vi "Page_AddCalSet.vi"(8 "error in (no error)":errorcluster, 11 "Configuration Paths":T1) -> (0 "error out":errorcluster, 3 "Configuration Paths out":T1)   [LabVIEW 2010]
uses:
  Config cluster.ctl
panel:
  in  "Delete Stim Profile":bool
  in  "Delete":bool
  in  "Selected Calibration Files":i32(listbox)
  in  "Add Calib":bool
  out "System Configuration File":string
  in  "Cancel Button":bool
  in  "OK Button":bool
  in  "Calibration files":i32[](listbox)
  # "1) Select the \"Calibration\" files for this calibration set"
  # "Available Calibration Files"
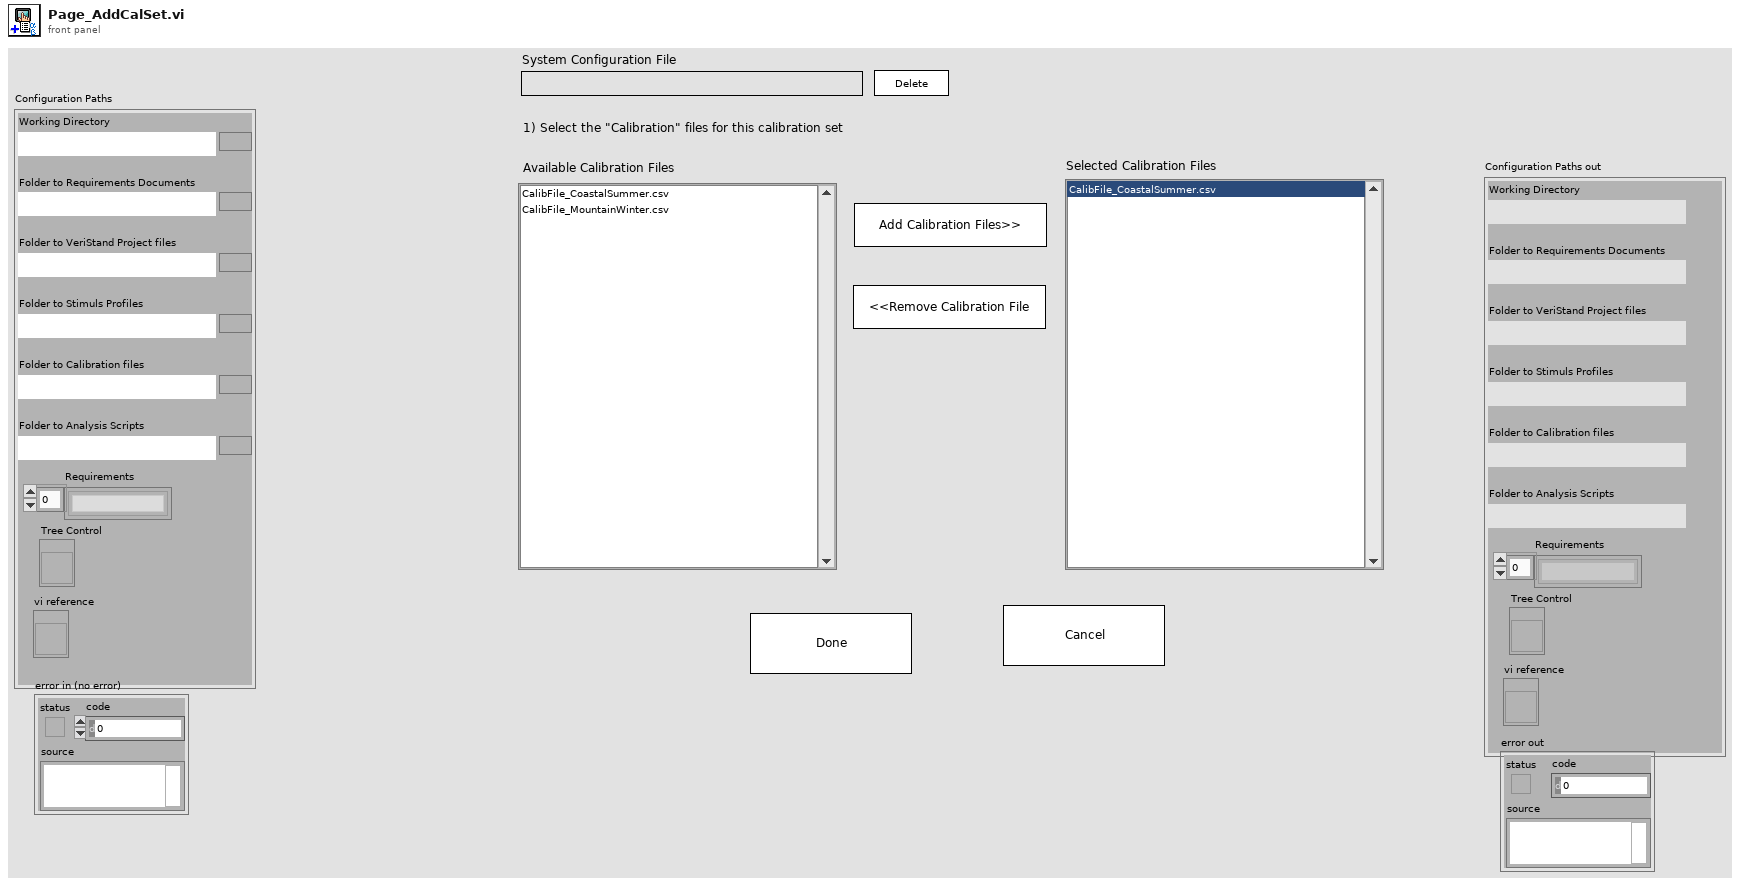
[diagram p1: front panel]
types:
  T1 = typedef "Config cluster.ctl" = cluster{"Working Directory":path, "Folder to Requirements Documents":path, "Folder to VeriStand Project files":path, "Folder to Stimuls Profiles":path, "Folder to Calibration files":path, "Folder to Analysis Scripts":path, "Requirements":string[], "Tree Control":refnum<vi>, "vi reference":refnum<vi>}
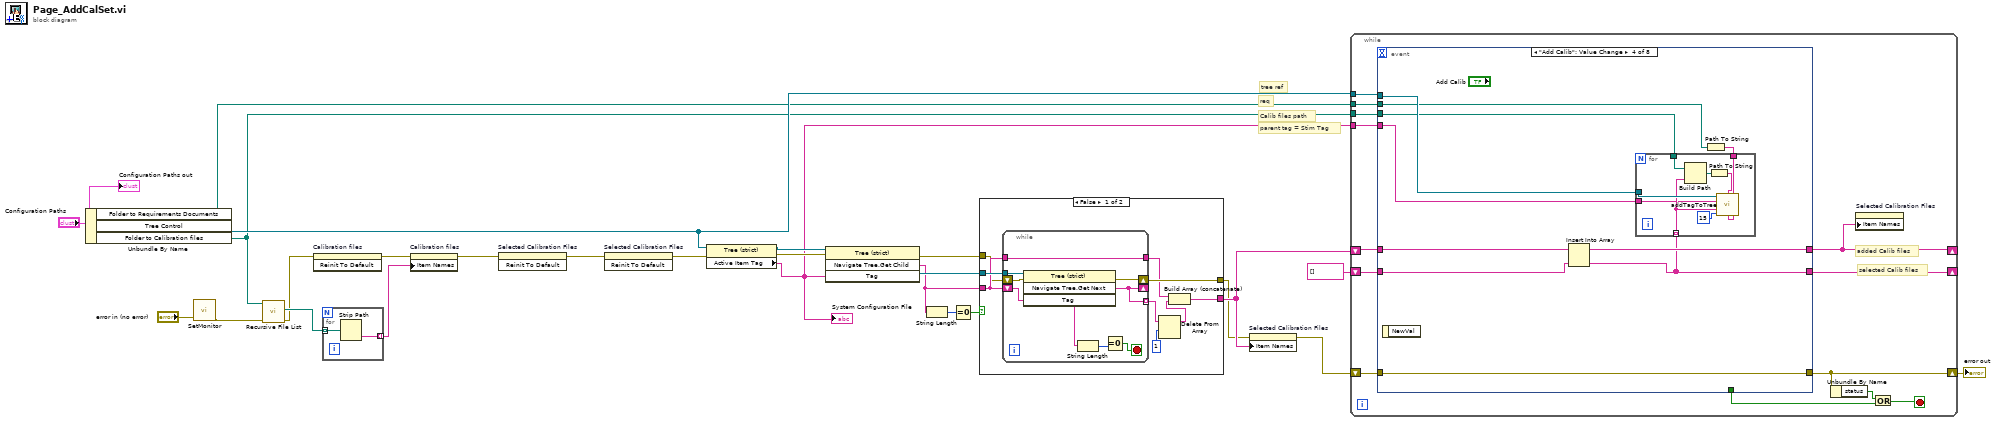
[diagram p0: block diagram]
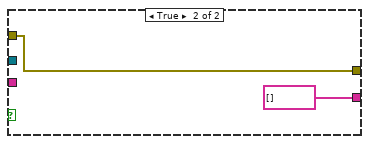
[diagram p2: hidden frame]
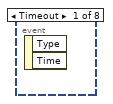
[diagram p3: hidden frame]
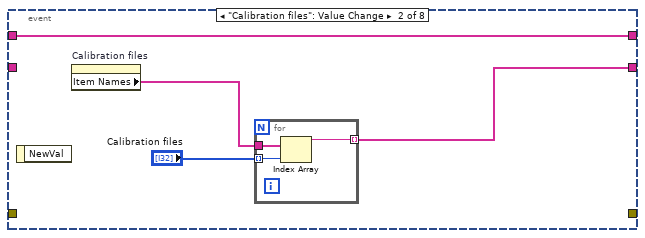
[diagram p4: hidden frame]
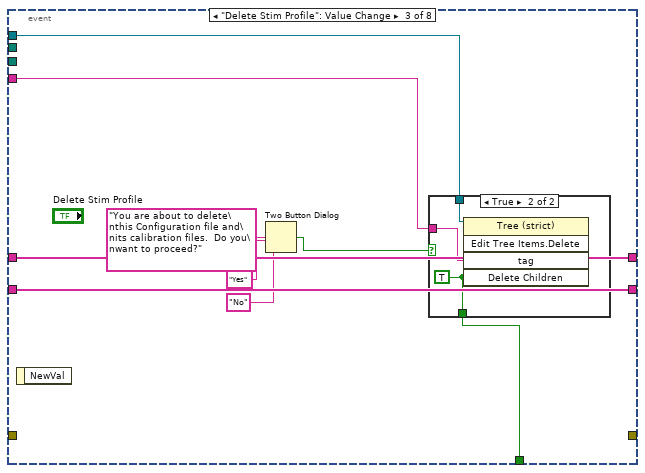
[diagram p5: hidden frame]
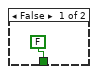
[diagram p6: hidden frame]
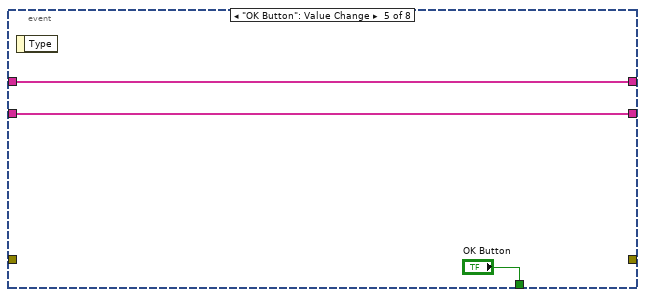
[diagram p7: hidden frame]
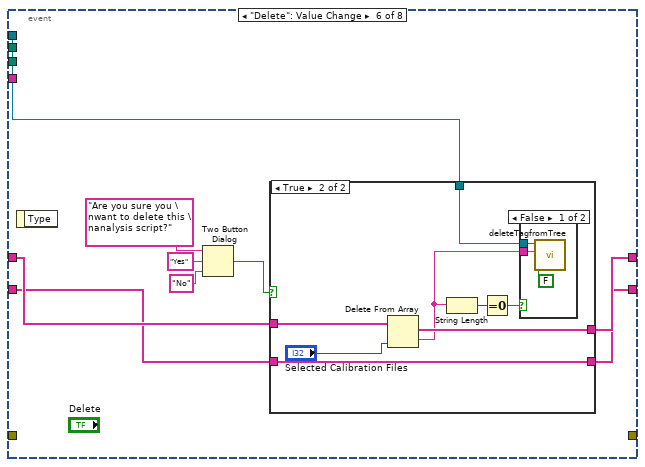
[diagram p8: hidden frame]
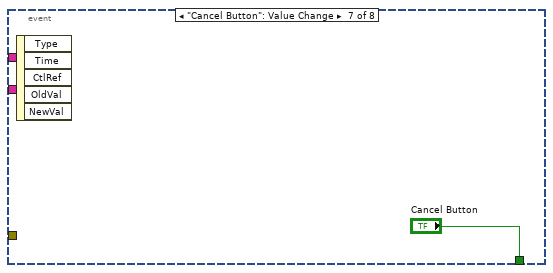
[diagram p11: hidden frame]
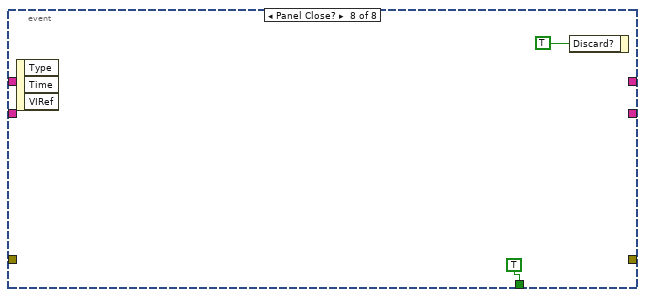
[diagram p12: hidden frame]
diagram:
  # "parent tag = Stim Tag"
  # "req"
  # "Calib files path"
  # "tree ref"
  n1 = Unbundle By Name("Configuration Paths") -> ("Folder to Requirements Documents"=w11:path, "Tree Control"=w13:refnum<vi>, "Folder to Calibration files"=w5:path)
  n2 = call "SetMonitor.vi"("error in (no error)"="error in (no error)") -> ("error out"=w1:errorcluster)  [unwired: 9 in, 1 out]
  n3 = call <vilib>:"Recursive File List.vi"("error in (no error)"=w1, "Folder Path"=w5) -> ("error out"=w4:errorcluster, "All Files in Dir"=w18:path[])  [unwired: 5 in, 3 out]
  n4 = invoke on="Calibration files" class="LstBox (strict)" method="Reinit To Default"(error in=w4) -> (error out=w20:errorcluster)  [unwired: 2 in, 2 out]
  n5 = for {
    tunnel: w18 -> [w28] mode=indexing
    tunnel: [w27] -> w17 mode=indexing
    n6 = Strip Path(path=w28) -> (name=w27:string)  [unwired: 1 out]
  }
  n7 = property on="Calibration files" class="LstBox (strict)"(error in=w20, "Item Names"=w17) -> (error out=w16:errorcluster)  [unwired: 1 in, 1 out]
  n8 = invoke on="Selected Calibration Files" class="LstBox (strict)" method="Reinit To Default"(error in=w16) -> (error out=w26:errorcluster)  [unwired: 2 in, 2 out]
  n9 = invoke on="Selected Calibration Files" class="LstBox (strict)" method="Reinit To Default"(error in=w26) -> (error out=w3:errorcluster)  [unwired: 2 in, 2 out]
  n10 = property class="Tree (strict)"(reference=w13, error in=w3) -> (reference out=w12:refnum<vi>, error out=w14:errorcluster, "Active Item Tag"=w7:string)
  "System Configuration File" <- w7
  n11 = invoke on="Invoke Node" class="Tree (strict)" method="Navigate Tree.Get Child"(reference=w12, error in=w14, "Tag"=w7) -> (reference out=w25:refnum<vi>, error out=w15:errorcluster, "Navigate Tree:Get Child"=w24:string)  [unwired: 1 in, 1 out]
  n12 = String Length(string=w24) -> (length=w23:i32)
  n13 = Equal To 0?(x=w23) -> (x = 0?=w22:bool)
  n14 = case shown="False" w22 {
    tunnel: [w37 w46] -> w10
    tunnel: w25 -> [w36 _]
    tunnel: [w33 string[] []] -> w21
    tunnel: w24 -> [w34 _]
    tunnel: w15 -> [w32 w46]
    frame False {
      n15 = while {
        shift-right: [w42] -> _
        shift-left: w34 -> [w41]
        tunnel: [w42] -> w31 mode=indexing
        tunnel: w36 -> [w40]
        tunnel: [w39] -> w35
        tunnel: w34 -> [w39]
        shift-right: [w43] -> w37
        shift-left: w32 -> [w38]
        stop <- w44 stop-if-true
        n16 = invoke on="Invoke Node" class="Tree (strict)" method="Navigate Tree.Get Next"(reference=w40, error in=w38, "Tag"=w41) -> (error out=w43:errorcluster, "Navigate Tree:Get Next Item"=w42:string)  [unwired: 1 in, 2 out]
        n17 = String Length(string=w42) -> (length=w45:i32)
        n18 = Equal To 0?(x=w45) -> (x = 0?=w44:bool)
      }
      n19 = Delete From Array(array=w31, length=1) -> (array with subset deleted=w30:string[])  [unwired: 1 in, 1 out]
      n20 = Build Array (concatenate)(w35, w30) -> (w33:string[])
    }
    frame True {
    }
  }
  n21 = property on="Selected Calibration Files" class="LstBox (strict)"(error in=w10, "Item Names"=w21) -> (error out=w9:errorcluster)  [unwired: 1 in, 1 out]
  n22 = while {
    shift-right: [w59] -> _
    shift-left: string[] [] -> [w58]
    shift-right: [w56] -> _
    shift-left: w21 -> [w57]
    tunnel: w13 -> [w55]
    tunnel: w11 -> [w54]
    tunnel: w5 -> [w60]
    shift-right: [w52] -> w8
    shift-left: w9 -> [w53]
    tunnel: w7 -> [w48]
    stop <- w49 stop-if-true
    # "added Calib files"
    # "selected Calib files"
    n23 = event shown="[3] \"Add Calib\": Value Change" {
      selector: _ -> [_ _ _ _ _ _ _ _]
      dyn-events: _ -> [_ _ _ _ _ _ _ _]
      timeout: _ -> [_ _ _ _ _ _ _ _]
      tunnel: w60 -> [_ _ _ w85 _ _ _ _]
      tunnel: [_ _ w70 _ "OK Button" _ "Cancel Button" TRUE ("Cancel Button")] -> w50
      tunnel: [_ w64 w75 w86 w99 w102 _ _] -> w59
      tunnel: w58 -> [_ _ w75 w86 w99 w103 _ _]
      tunnel: w57 -> [_ w63 w76 w89 w98 w109 _ _]
      tunnel: [_ w63 w76 w87 w98 w108 _ _] -> w56
      tunnel: w55 -> [_ _ w71 w88 _ w107 _ _]
      tunnel: w54 -> [_ _ _ w84 _ _ _ _]
      tunnel: w53 -> [_ _ _ w82 _ _ _ _]
      tunnel: [_ _ _ w82 _ _ _ _] -> w52
      tunnel: w48 -> [_ _ w68 w81 _ _ _ _]
      event Timeout {
        n24 = event-data() -> ()  [unwired: 1 in, 2 out]
      }
      event "Calibration files": Value Change {
        n25 = event-data() -> ()  [unwired: 1 in, 1 out]
        n26 = property on="Calibration files" class="LstBox (strict)"() -> ("Item Names"=w61:string[])  [unwired: 2 in, 2 out]
        n27 = for {
          tunnel: [w67] -> w64 mode=indexing
          tunnel: w61 -> [w66]
          tunnel: "Calibration files" -> [w65] mode=indexing
          n28 = Index Array(array=w66, index=w65) -> (element=w67:string)
        }
      }
      event "Delete Stim Profile": Value Change {
        n29 = event-data() -> ()  [unwired: 1 in, 1 out]
        n30 = Two Button Dialog(message="You are about to delete\nthis Configuration file and\nits calibration files.  Do you\nwant to proceed?", 1:"No" ("F button name (\"Cancel\")"), 2:"Yes" ("T button name (\"OK\")")) -> (T button?=w69:bool)
        n31 = case shown="True" w69 {
          tunnel: w71 -> [_ w80]
          tunnel: [FALSE ("Delete Children?") w79] -> w70
          tunnel: w68 -> [_ w78]
          frame False {
          }
          frame True {
            w79 = TRUE ("Delete Children?")
            n32 = invoke on="Invoke Node" class="Tree (strict)" method="Edit Tree Items.Delete"(reference=w80, "tag"=w78, "Delete Children"=w79) -> ()  [unwired: 2 in, 5 out]
          }
        }
      }
      event "Add Calib": Value Change {
        n33 = event-data() -> ()  [unwired: 1 in, 1 out]
        n34 = Insert Into Array(array=w89, new element=w86) -> (w87:string[])  [unwired: 1 in]
        n35 = Path To String(path=w84) -> (string=w83:string)
        n36 = for {
          tunnel: w88 -> [w97]
          tunnel: w86 -> [w95] mode=indexing
          tunnel: w85 -> [w94]
          tunnel: w83 -> [w92]
          tunnel: w81 -> [w91]
          n37 = Build Path(base path=w94, name or relative path=w95) -> (appended path=w93:path)
          n38 = Path To String(path=w93) -> (string=w90:string)
          n39 = call "addTagToTree.vi"("Tree ref"=w97, "Calibration path"=w90, "parent tag"=w91, "new tag"=w95, "Symbol"=15, "Req doc path"=w92) -> ()  [unwired: 9 in, 1 out]
        }
      }
      event "OK Button": Value Change {
        n40 = event-data() -> ()  [unwired: 1 in, 1 out]
      }
      event "Delete": Value Change {
        n41 = event-data() -> ()  [unwired: 1 in, 1 out]
        n42 = Two Button Dialog(message="Are you sure you \nwant to delete this \nanalysis script?", 1:"No" ("F button name (\"Cancel\")"), 2:"Yes" ("T button name (\"OK\")")) -> (T button?=w101:bool)
        n43 = case shown="True" w101 {
          tunnel: w109 -> [w111 w118]
          tunnel: [w111 w117] -> w108
          tunnel: w107 -> [_ w116]
          tunnel: w103 -> [w110 w115]
          tunnel: [w110 w115] -> w102
          frame False {
          }
          frame True {
            n44 = Delete From Array(array=w118, index="Selected Calibration Files") -> (deleted portion=w114:string, array with subset deleted=w117:string[])  [unwired: 1 in]
            n45 = String Length(string=w114) -> (length=w113:i32)
            n46 = Equal To 0?(x=w113) -> (x = 0?=w112:bool)
            n47 = case shown="False" w112 {
              tunnel: w116 -> [w122 _]
              tunnel: w114 -> [w120 _]
              frame False {
                n48 = call "deleteTagfromTree.vi"("Delete Children?"=FALSE, "Tag"=w120, "Tree Ref"=w122) -> ()  [unwired: 7 in, 2 out]
              }
              frame True {
              }
            }
          }
        }
      }
      event "Cancel Button": Value Change {
        n49 = event-data() -> ()  [unwired: 1 in, 5 out]
      }
      event Panel Close? {
        n50 = event-data() -> ()  [unwired: 1 in, 3 out]
        n51 = event-data("Discard?"=TRUE) -> ()  [unwired: 1 in, 1 out]
      }
    }
    n52 = Unbundle By Name(w52) -> ("status"=w51:bool)
    n53 = property on="Selected Calibration Files" class="LstBox (strict)"("Item Names"=w56) -> ()  [unwired: 2 in, 2 out]
    n54 = Or(x=w51, y=w50) -> (x .or. y?=w49:bool)
  }
  "error out" <- w8
  "Configuration Paths out" <- "Configuration Paths"
